vi "Ref Mem.vi"() -> ()   [LabVIEW 2010]
uses:
  <vilib>/Platform/TimedLoop/XDataNode/XDataNode.xnode
  <vilib>/Platform/TimedLoop/XDataNode/timing_clust.ctl
  <vilib>/Platform/TimedLoop/XDataNode/nitl_modes.ctl
  <vilib>/Platform/TimedLoop/XDataNode/wakeup.ctl
  <vilib>/DAQmx/write.llb/DAQmx Write (Analog DBL 1Chan 1Samp).vi
  <vilib>/DAQmx/create/channels.llb/DAQmx Create Channel (AO-Voltage-Basic).vi
  <vilib>/DAQmx/configure/timing.llb/DAQmx Timing (Sample Clock).vi
  <vilib>/xnet/xnet.llb/XNET Read (State FlexRay Cycle Macrotick).vi
  <vilib>/xnet/xnet.llb/XNET Write (Signal Single-point).vi
  <vilib>/xnet/xnet.llb/XNET Read (Signal Single-point).vi
  <vilib>/daqmx/miscellaneous.llb/DAQmx Fill In Error Info.vi
  <vilib>/Platform/TimedLoop/XDataNode/XDNodeRunTimeDep.lvlib
panel:
  in  "Select":bool caption="Each VI running needs this switch set different!"
  out "Input Data":dbl
  in  "Output Data":dbl
  out "dt":u32=275
  out "error out":errorcluster
  in  "stop":bool
  # "VI1: set high\nVI2: set low"
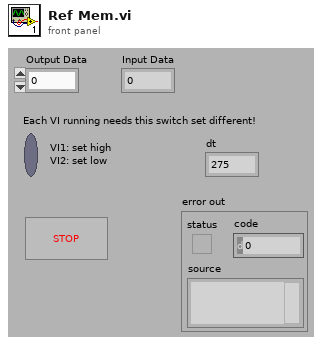
[diagram p1: front panel]
types:
  T1 = typedef "Sessions.ctl" = cluster{"In":refnum<k21>, "Out":refnum<k21>, "NIT Start":u32}
  T2 = typedef "XDNodeRunTimeDep.lvlib/timing_clust.ctl" = cluster{"Expected End [f-1]":u64, "Actual End [f-1]":u64, "Finished Late? [f-1]":bool, "Expected End [i-1]":u64, "Actual End [i-1]":u64, "Finished Late? [i-1]":bool, "Expected Start [i]":u64, "Actual Start [i]":u64, "Expected Start [f]":u64, "Actual Start [f]":u64, "Source Name":string, "Structure Name":string, "Period":i64, "Deadline":i64, "Offset":i64, "Start":i64, "Priority":i32, "Timeout":i32, "Mode":T3, "Wakeup Reason":T4, "Error":errorcluster, "Source Type":string, "Secondary Source Type":string, "Global End Time":u64, "Global Start Time":u64, "Frame Duration":u64, "Iteration Duration":u64, "Assigned CPU":i32, "I/O Scan Engine Mode":u32}
  T3 = typedef "XDNodeRunTimeDep.lvlib/nitl_modes.ctl" = enum32{"No Change", "Process missed periods, maintain original phase", "Discard missed periods, maintain original phase", "Process missed periods, ignore original phase", "Discard missed periods, ignore original phase"}
  T4 = typedef "XDNodeRunTimeDep.lvlib/wakeup.ctl" = enum32{"Normal", "Aborted", "Asynchronous wakeup", "Timing source error", "Timed loop error", "Timeout"}
  T5 = typedef "2 States Action.ctl" = enum16{"FR Write", "FR Read and DAQ Write", "None"}
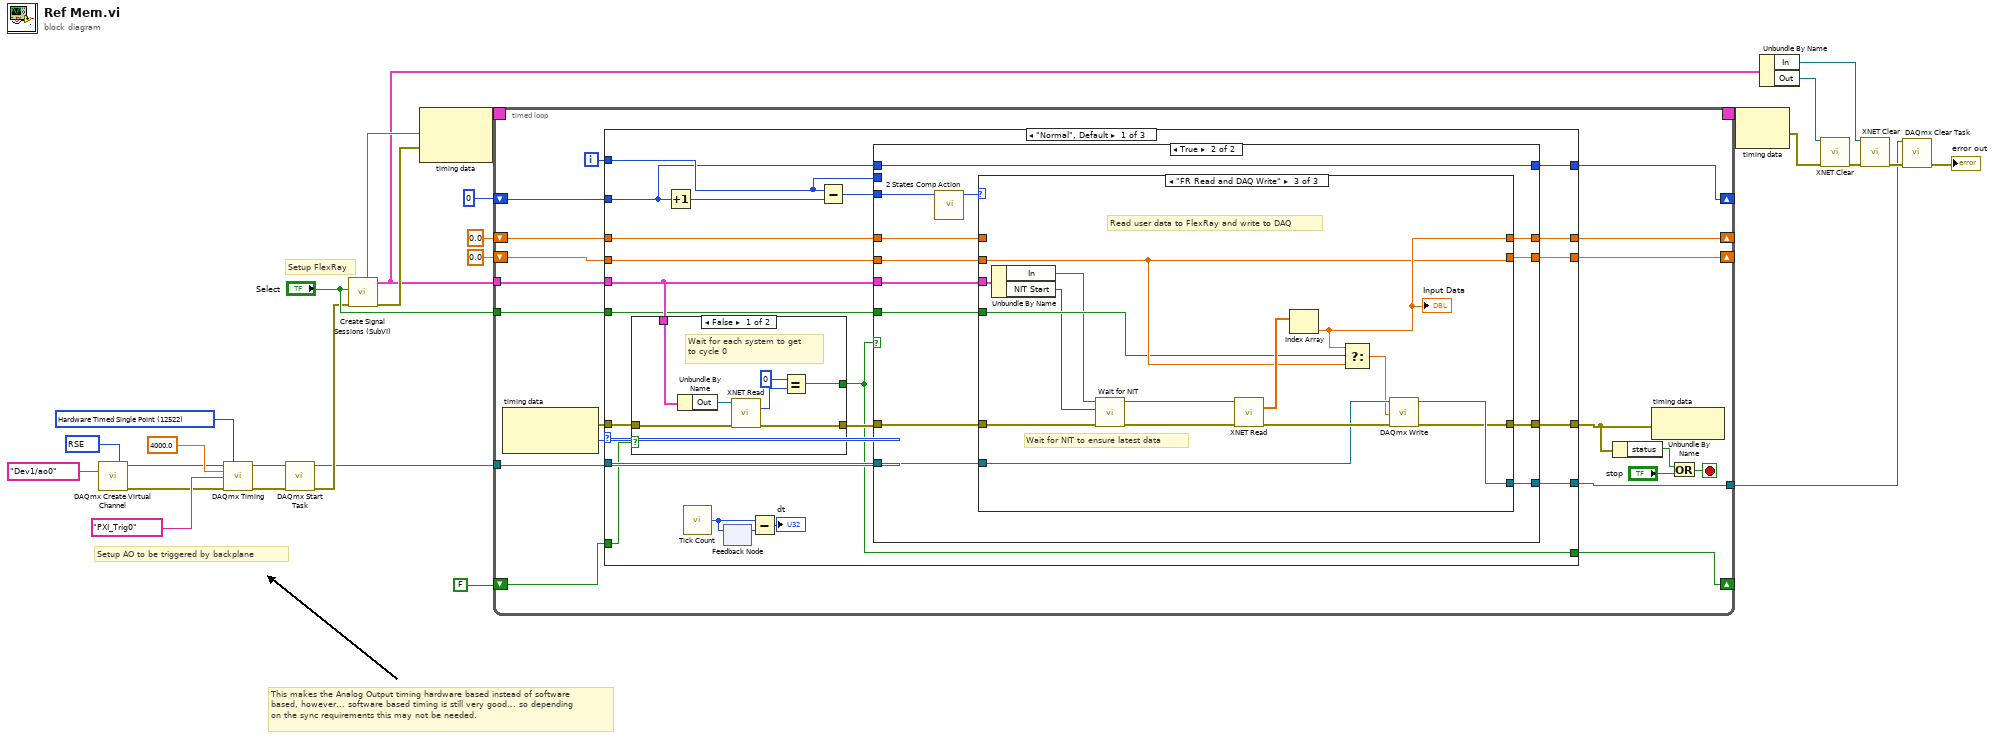
[diagram p0: block diagram]
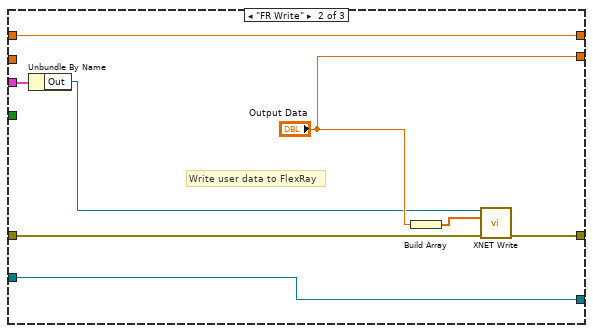
[diagram p5: hidden frame]
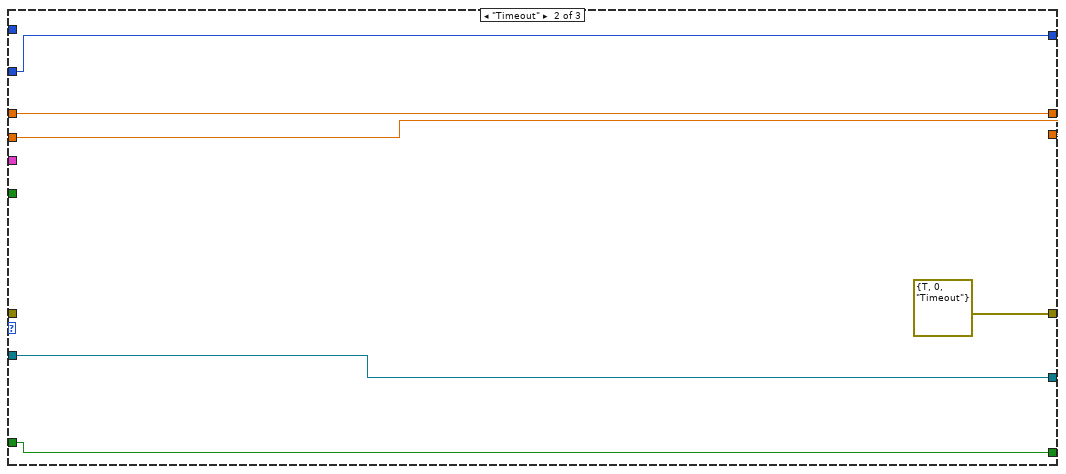
[diagram p6: hidden frame]
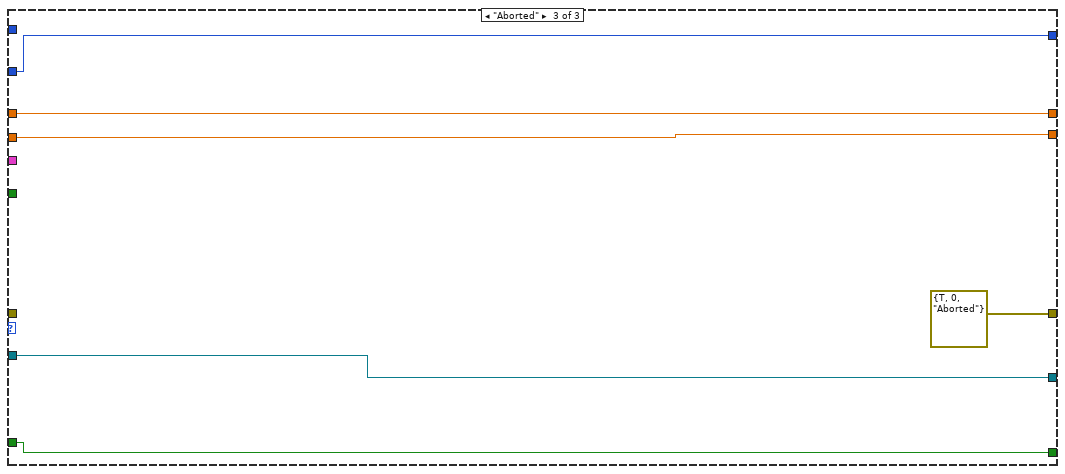
[diagram p7: hidden frame]
diagram:
  w9 = 12522 items=["Finite Samples"=10178, "Continuous Samples"=10123, "Hardware Timed Single Point"=12522] ("sample mode")
  w11 = 10083 items=["Default"=-1, "RSE"=10083, "Differential"=10106, "Pseudodifferential"=12529] ("output terminal configuration")
  # "Setup FlexRay"
  # "This makes the Analog Output timing hardware based instead of software based, however... software based timing is still very good... so depending on the sync requirements this may not be needed."
  # "Setup AO to be triggered by backplane"
  n1 = call-poly <vilib>:"DAQmx Create Virtual Channel.vi"("output terminal configuration"=w11, "physical channels"=tag "Dev1/ao0") -> ("task out"=w5:refnum<k21>, "error out"=w6:errorcluster)  [unwired: 12 in]
  n2 = call-poly <vilib>:"DAQmx Timing.vi"("task/channels in"=w5, "sample mode"=w9, "rate"=4000.0, "source"=tag "PXI_Trig0", "error in"=w6) -> ("task out"=w3:refnum<k21>, "error out"=w4:errorcluster)  [unwired: 9 in]
  n3 = call <vilib>:"DAQmx Start Task.vi"("task/channels in"=w3, "error in"=w4) -> ("task out"=w1:refnum<k21>, "error out"=w2:errorcluster)  [unwired: 12 in]
  n4 = call "Create Signal Sessions (SubVI).vi"("error in"=w2, "Select"="Select") -> ("error out"=w17:errorcluster, "Sessions"=w15:T1, "timing source out"=w16:string)  [unwired: 7 in]
  n5 = node-c288(w16, w17) -> (w28:T2)
  n6 = timed-loop {
    timing: w28 -> [_]
    timing-out: [_] -> w27
    shift-right: [w43] -> _
    shift-left: 0.0 ("element") -> [w45]
    shift-right: [w44] -> _
    shift-left: 0.0 ("element") -> [w46]
    tunnel: w1 -> [w42]
    tunnel: [w41] -> w23
    shift-right: [w31] -> _
    shift-left: 0 -> [w33]
    shift-right: [w34] -> _
    shift-left: FALSE -> [w35]
    tunnel: w15 -> [w30]
    tunnel: "Select" -> [w29]
    i -> [w32]
    stop <- w37 stop-if-true
    n7 = node-c288() -> (w36:errorcluster, w47:T4)  [unwired: 1 in]
    n8 = case shown="\"Normal\", Default" w47 {
      tunnel: w36 -> [w61 _ _]
      tunnel: [w64 errorcluster {"status"=TRUE, "code"=0, "source"="Timeout"} ("Error") errorcluster {"status"=TRUE, "code"=0, "source"="Aborted"} ("Error")] -> w38
      tunnel: w46 -> [w68 w127 w133]
      tunnel: w45 -> [w67 w126 w132]
      tunnel: [w66 w127 w133] -> w44
      tunnel: [w65 w126 w132] -> w43
      tunnel: w42 -> [w63 w125 w131]
      tunnel: [w62 w125 w131] -> w41
      tunnel: w35 -> [w59 w124 w130]
      tunnel: [w58 w124 w130] -> w34
      tunnel: w33 -> [w51 w123 w129]
      tunnel: w32 -> [w52 _ _]
      tunnel: [w50 w123 w129] -> w31
      tunnel: w30 -> [w49 _ _]
      tunnel: w29 -> [w48 _ _]
      frame "Normal", Default {
        n9 = case shown="False" w59 {
          selector: w59 -> [_ w76]
          tunnel: w61 -> [w75 w77]
          tunnel: [w74 w77] -> w60
          tunnel: [w72 w76] -> w58
          tunnel: w49 -> [w71 _]
          frame False {
            # "Wait for each system to get\nto cycle 0"
            n10 = Unbundle By Name(w71) -> ("Out"=w70:refnum<k21>)
            n11 = call-poly <vilib>:"XNET Read.vi"("session in"=w70, "error in (no error)"=w75) -> ("cycle"=w73:u8, "error out"=w74:errorcluster)  [unwired: 10 in, 2 out]
            n12 = Equal?(x=u8 0, y=w73) -> (x = y?=w72:bool)
          }
          frame True {
          }
        }
        n13 = Increment(x=w51) -> (x+1=w54:i32)
        n14 = call "Tick Count"() -> ("Tick Count(uSec)"=w56:u32)
        n15 = feedback #1() -> (w57:u32)  [unwired: 1 in]
        n16 = feedback-in #1(w56) -> ()
        n17 = Subtract(x=w56, y=w57) -> (x-y=→"dt":u32)
        n18 = Subtract(x=w52, y=w54) -> (x-y=w53:i32)
        n19 = case shown="True" w58 {
          tunnel: w53 -> [_ w95]
          tunnel: w68 -> [w80 w93]
          tunnel: w60 -> [w79 w92]
          tunnel: w67 -> [w81 w91]
          tunnel: [w80 w90] -> w66
          tunnel: [w81 w89] -> w65
          tunnel: [w79 w88] -> w64
          tunnel: w63 -> [w78 w87]
          tunnel: [w78 w86] -> w62
          tunnel: w52 -> [w82 _]
          tunnel: w51 -> [_ w85]
          tunnel: [w82 w85] -> w50
          tunnel: w49 -> [_ w84]
          tunnel: w48 -> [_ w83]
          frame False {
            # "Still waiting for cycles on each target to sync to 0."
          }
          frame True {
            n20 = call "2 States Comp Action.vi"("Iteration"=w95) -> ("Action"=w94:T5)  [unwired: 10 in]
            n21 = case shown="\"FR Read and DAQ Write\"" w94 {
              tunnel: w93 -> [w97 _ w115]
              tunnel: w92 -> [w96 w107 w111]
              tunnel: [w96 w106 w118] -> w88
              tunnel: w91 -> [w98 w105 _]
              tunnel: [w97 "Output Data" w115] -> w90
              tunnel: [w98 w105 w116] -> w89
              tunnel: w87 -> [w99 w104 w120]
              tunnel: [w99 w104 w119] -> w86
              tunnel: w84 -> [_ w101 w114]
              tunnel: w83 -> [_ _ w113]
              frame "None", Default {
              }
              frame "FR Write" {
                # "Write user data to FlexRay"
                n22 = Unbundle By Name(w101) -> ("Out"=w100:refnum<k21>)
                n23 = Build Array("Output Data") -> (w103:dbl[])
                n24 = call-poly <vilib>:"XNET Write.vi"("session in"=w100, "data"=w103, "error in (no error)"=w107) -> ("error out"=w106:errorcluster)  [unwired: 11 in, 1 out]
              }
              frame "FR Read and DAQ Write" {
                # "Wait for NIT to ensure latest data"
                # "Read user data to FlexRay and write to DAQ"
                n25 = Unbundle By Name(w114) -> ("In"=w110:refnum<k21>, "NIT Start"=w108:u32)
                n26 = call "Wait for NIT.vi"("Error"=w111, "NIT Start"=w108, "session in"=w110) -> ("Error out"=w112:errorcluster, "session out"=w109:refnum<k21>)  [unwired: 7 in]
                n27 = call-poly <vilib>:"XNET Read.vi"("session in"=w109, "error in (no error)"=w112) -> ("data"=w122:dbl[], "error out"=w121:errorcluster)  [unwired: 11 in, 1 out]
                n28 = Index Array(array=w122) -> (element=w116:dbl)  [unwired: 1 in]
                "Input Data" <- w116
                n29 = Select(t=w116, s=w113, f=w115) -> (s? t:f=w117:dbl)
                n30 = call-poly <vilib>:"DAQmx Write.vi"("task/channels in"=w120, "data"=w117, "error in"=w121) -> ("task out"=w119:refnum<k21>, "error out"=w118:errorcluster)  [unwired: 10 in, 1 out]
              }
            }
          }
        }
      }
      frame "Timeout" {
      }
      frame "Aborted" {
      }
    }
    n31 = Unbundle By Name(w38) -> ("status"=w39:bool)
    n32 = node-c288(w38) -> ()  [unwired: 1 out]
    n33 = Or(x=w39, y="stop") -> (x .or. y?=w37:bool)
  }
  n34 = node-c288(w27) -> (w26:errorcluster)
  n35 = Unbundle By Name(w15) -> ("In"=w13:refnum<k21>, "Out"=w14:refnum<k21>)
  n36 = call <vilib>:"XNET Clear.vi"("session in"=w14, "error in (no error)"=w26) -> ("error out"=w25:errorcluster)  [unwired: 13 in]
  n37 = call <vilib>:"XNET Clear.vi"("session in"=w13, "error in (no error)"=w25) -> ("error out"=w24:errorcluster)  [unwired: 13 in]
  n38 = call <vilib>:"DAQmx Clear Task.vi"("task in"=w23, "error in"=w24) -> ("error out"=→"error out":errorcluster)  [unwired: 13 in]
